vi "call dll example.vi"() -> ()   [LabVIEW 2015]
uses:
  build/PwrXtalCal.dll
panel:
  out "result":dbl
  in  "Freq":dbl=5180000000.0
  in  "RL":dbl
  in  "PhyPort":u16=6
  in  "PwrFreq":u16
  in  "VISA Resource Name":string="TCPIP0::10.144.41.48::inst0::INSTR"
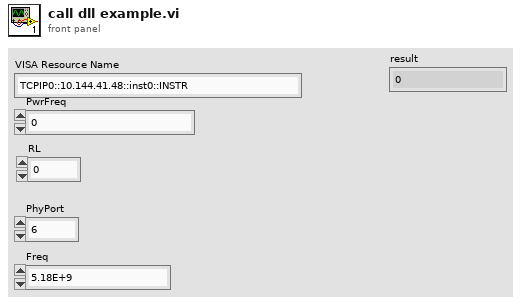
[diagram p1: front panel]
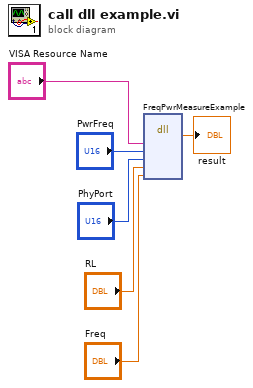
[diagram p0: block diagram]
diagram:
  n1 = dll-call lib="C:/Users/Mingming Yang/Documents/GitHub/PwrXtalCalDLL/build/PwrXtalCal.dll" fn="FreqPwrMeasureExample"("VISA Resource Name"="VISA Resource Name", "PwrFreq"="PwrFreq", "PhyPort"="PhyPort", "RL"="RL", "Freq"="Freq") -> ("result"=→"result":dbl)  [unwired: 8 in, 2 out]
